vi "FrontMostVI.vi"(0 "VI Reference In":refnum<vi>, 7 "Front Panel Window:Is Frontmost(T)":bool=TRUE, 11 "error in":errorcluster) -> (4 "VI Reference Out":refnum<vi>, 15 "error out":errorcluster)   [LabVIEW 2016, in "Drona.lvlib"]
doc: "Makes the front panel of the VI to frontmost, given the VI reference"
uses:
  Drona.lvlib
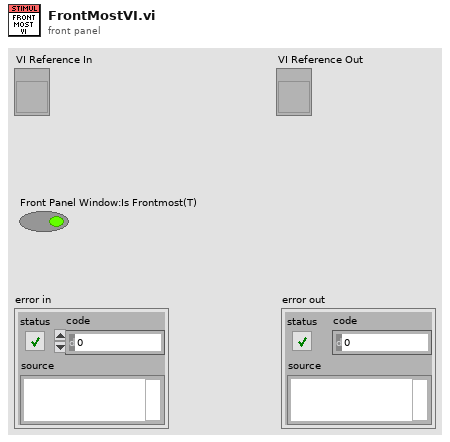
[diagram p1: front panel]
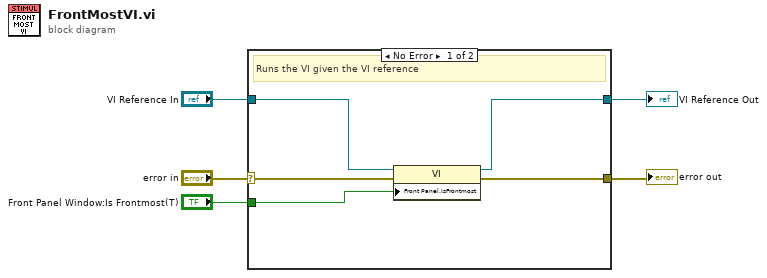
[diagram p0: block diagram]
diagram:
  n1 = case shown="No Error" "error in" {
    selector: "error in" -> [w10 w12]
    tunnel: "VI Reference In" -> [w7 w11]
    tunnel: [w8 w11] -> w3
    tunnel: [w9 w12] -> w2
    tunnel: "Front Panel Window:Is Frontmost(T)" -> [w6 _]
    frame No Error {
      # "Runs the VI given the VI reference"
      n2 = property class="VI"(reference=w7, error in=w10, "Front Panel.IsFrontmost"=w6) -> (reference out=w8:refnum<vi>, error out=w9:errorcluster)
    }
    frame Error {
    }
  }
  "error out" <- w2
  "VI Reference Out" <- w3
